vi "Drive Controller.vi"(8 "error in":errorcluster) -> ()   [LabVIEW 2019]
doc: "This VI executes continuously carrying out the current operation and responding to updates or new operation requests. It will often contain the timing or control code that is difficult to place directly in TeleOp. This VI generally opens all sensors and motors and isolates the rest of the robot code from knowing implementation details of how the operations are carried out."
uses:
  <vilib>/Rock Robotics/WPI/Framework/Completion Status.ctl
  Drive Setpoints.ctl
  Drive Operations.ctl
  <vilib>/Rock Robotics/WPI/ThirdParty/Phoenix-LabVIEW/Motor Controller/Controls/CTRE_Phoenix_MotorControl_ControlMode.ctl
  <vilib>/Rock Robotics/WPI/ThirdParty/Phoenix-LabVIEW/Motor Controller/Get/CTRE_Phoenix_MotorController_GetQuadratureData.vi
  <vilib>/Rock Robotics/WPI/SafetyOutput/WPI_SafetyOutputConfigMenu.ctl
  <vilib>/Rock Robotics/WPI/ThirdParty/Phoenix-LabVIEW/Motor Controller/Get/CTRE_Phoenix_MotorController_GetSelectedSensorData.vi
  <vilib>/Rock Robotics/WPI/RobotDrive/WPI_RobotDriveOpen2MotorWithExistingMotors.vi
panel:
  out "Analog Position 2":dbl
  out "Iterations":i32
  out "Analog Position":dbl
  in  "Interactive Values":T1
  in  "Buttons":cluster{"Execute Cmd":bool, "Abort Cmd":bool}
  out "Command Timing":cluster{"Start Time (ms)":u32, "Iterations":i32}
  out "Status":T3
  out "Current\nCmd":string
  # "Tip: The graph shows the motor setpoints. It may also be helpful to observe inputs and sensor values.\nYou may also want to display tuning or debugging controls."
  # "Interactive Command: You may fill in the settings for a command\nand schedule it with the Execute button. You can observe and abort\nany command while fine tuning the code for the controller."
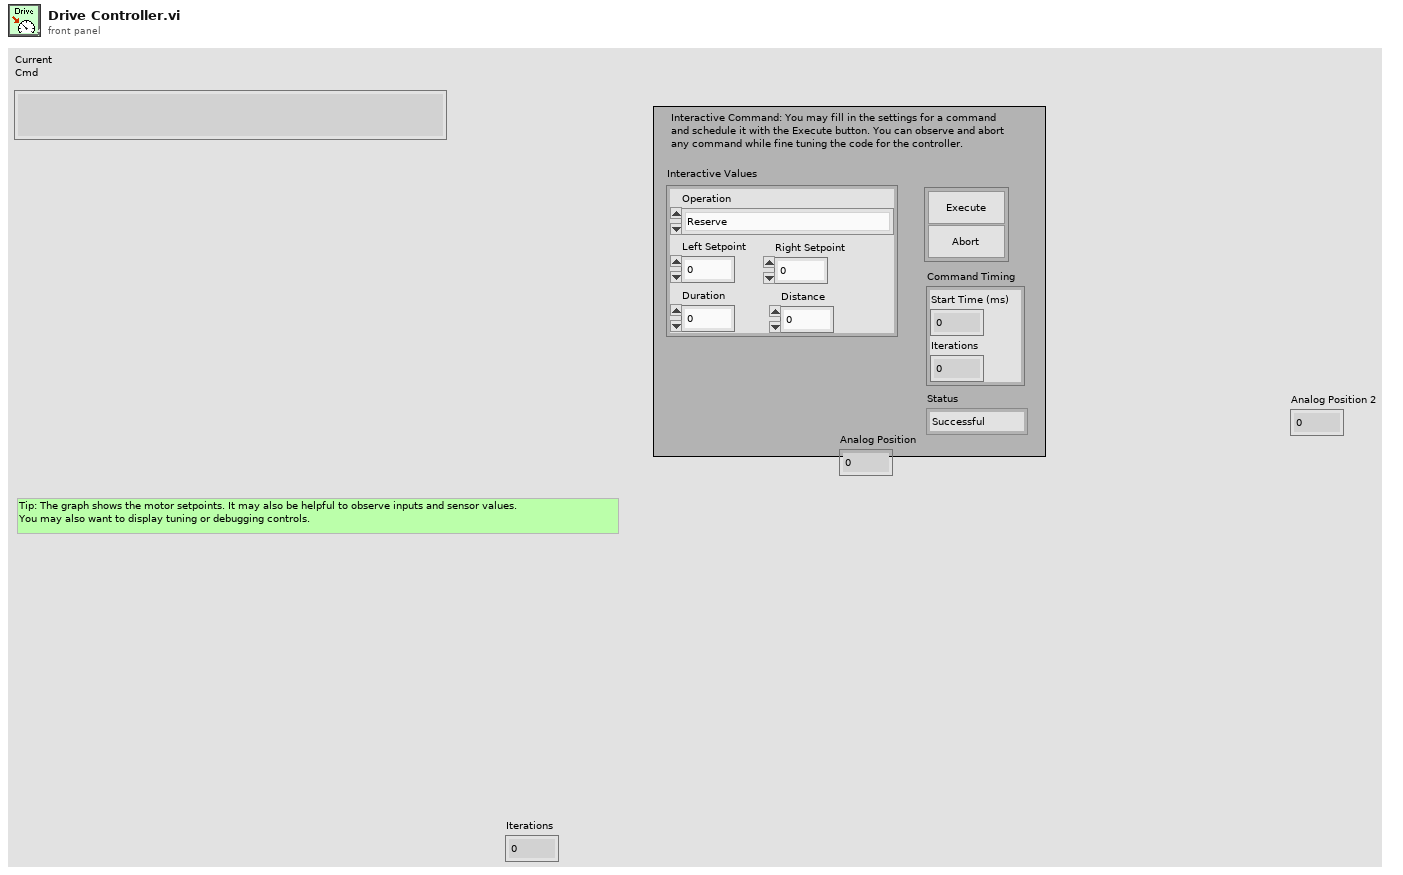
[diagram p1: front panel]
types:
  T1 = typedef "Drive Setpoints.ctl" = cluster{"Operation":T2, "Left Setpoint":dbl, "Right Setpoint":dbl, "Duration":dbl, "Distance":dbl}
  T2 = typedef "Drive Operations.ctl" = enum16{"Reserve", "Read Current", "Immediate", "Drive for Time", "Drive for Distance", "Turn angle"}
  T3 = typedef "Completion Status.ctl" = enum16{"Successful", "Aborted", "Incomplete"}
  T4 = typedef "WPI_SafetyOutputConfigMenu.ctl" = enum16{"Enable", "Disable"}
  T5 = typedef "WPI_MotorControlDeviceRef.ctl" = cluster{"DeviceStatus":errorcluster, "Type":T6, "PWM":cluster{"PWM Channel":T7, "DeadBand":T8}, "CAN":cluster{"Device Number":u8, "SetOutput VI Ref":variant, "GetOutput VI Ref":variant, "Enable VI Ref":variant, "Disable VI Ref":variant, "Data":variant}, "Invert":bool, "DIO PWM":cluster{"PWM \"Enable\" Channel":T7, "DIOChannel":T9, "PWM Rate":dbl}}
  T6 = typedef "WPI_MotorControlType.ctl" = enum16{"PWM", "CAN", "DIO PWM"}
  T7 = typedef "FPGA_DIOPWMChannel.ctl" = enum8{"PWM 0", "PWM 1", "PWM 2", "PWM 3", "PWM 4", "PWM 5", "PWM 6", "PWM 7", "PWM 8", "PWM 9", "PWM MXP 0", "PWM MXP 1", "PWM MXP 2", "PWM MXP 3", "PWM MXP 4", "PWM MXP 5", "PWM MXP 6", "PWM MXP 7", "PWM MXP 8", "PWM MXP 9", "Invalid"}
  T8 = typedef "WPI_PWMDeadband.ctl" = cluster{"Name":string, "maxPositivePwm":i32, "minPositivePwm":i32, "centerPwm":i32, "maxNegativePwm":i32, "minNegativePwm":i32, "angularRange":u16}
  T9 = typedef "FPGA_DIOChannel.ctl" = enum8{"DIO 0", "DIO 1", "DIO 2", "DIO 3", "DIO 4", "DIO 5", "DIO 6", "DIO 7", "DIO 8", "DIO 9", "DIO MXP 0", "DIO MXP 1", "DIO MXP 2", "DIO MXP 3", "DIO MXP 4", "DIO MXP 5", "DIO MXP 6", "DIO MXP 7", "DIO MXP 8", "DIO MXP 9", "DIO MXP 10", "DIO MXP 11", "DIO MXP 12", "DIO MXP 13", "DIO MXP 14", "DIO MXP 15", "SPI Port CS1", "SPI Port CS2", "SPI Port CS3", "SPI Port MISO", "SPI Port MOSI", "Invalid"}
  T10 = typedef "WPI_RobotDriveDevRef.ctl" = cluster{"DevStatus":errorcluster, "Motors[]":T5[], "Square Inputs":bool, "Max Output":dbl}
  T11 = enum16{"FollowerType_PercentOutput", "FollowerType_AuxOutput1"}
  T12 = typedef "Command Status Info.ctl" = cluster{"Name":string, "Status":T3, "notifier out":T13}
  T13 = typedef "Completion Notifier.ctl" = refnum<notifier>
  T14 = cluster{"SubSystem Data":T1, cluster{"Start Time (ms)":u32, "Iterations":i32}, cluster{"Command Info":T12, "Description":string, "Default Command":T1, "queue out":refnum<queue>, "Subsystem Name":string}}
  T15 = typedef "CTRE_Phoenix_MotorControl_ControlMode.ctl" = u16
  T16 = cluster{"SubSystem Data":T1, cluster{"Start Time (ms)":u32, "Iterations":i32}, "Default Command Arguments":cluster{"Command Info":T12, "Description":string, "Default Command":T1, "queue out":refnum<queue>, "Subsystem Name":string}}
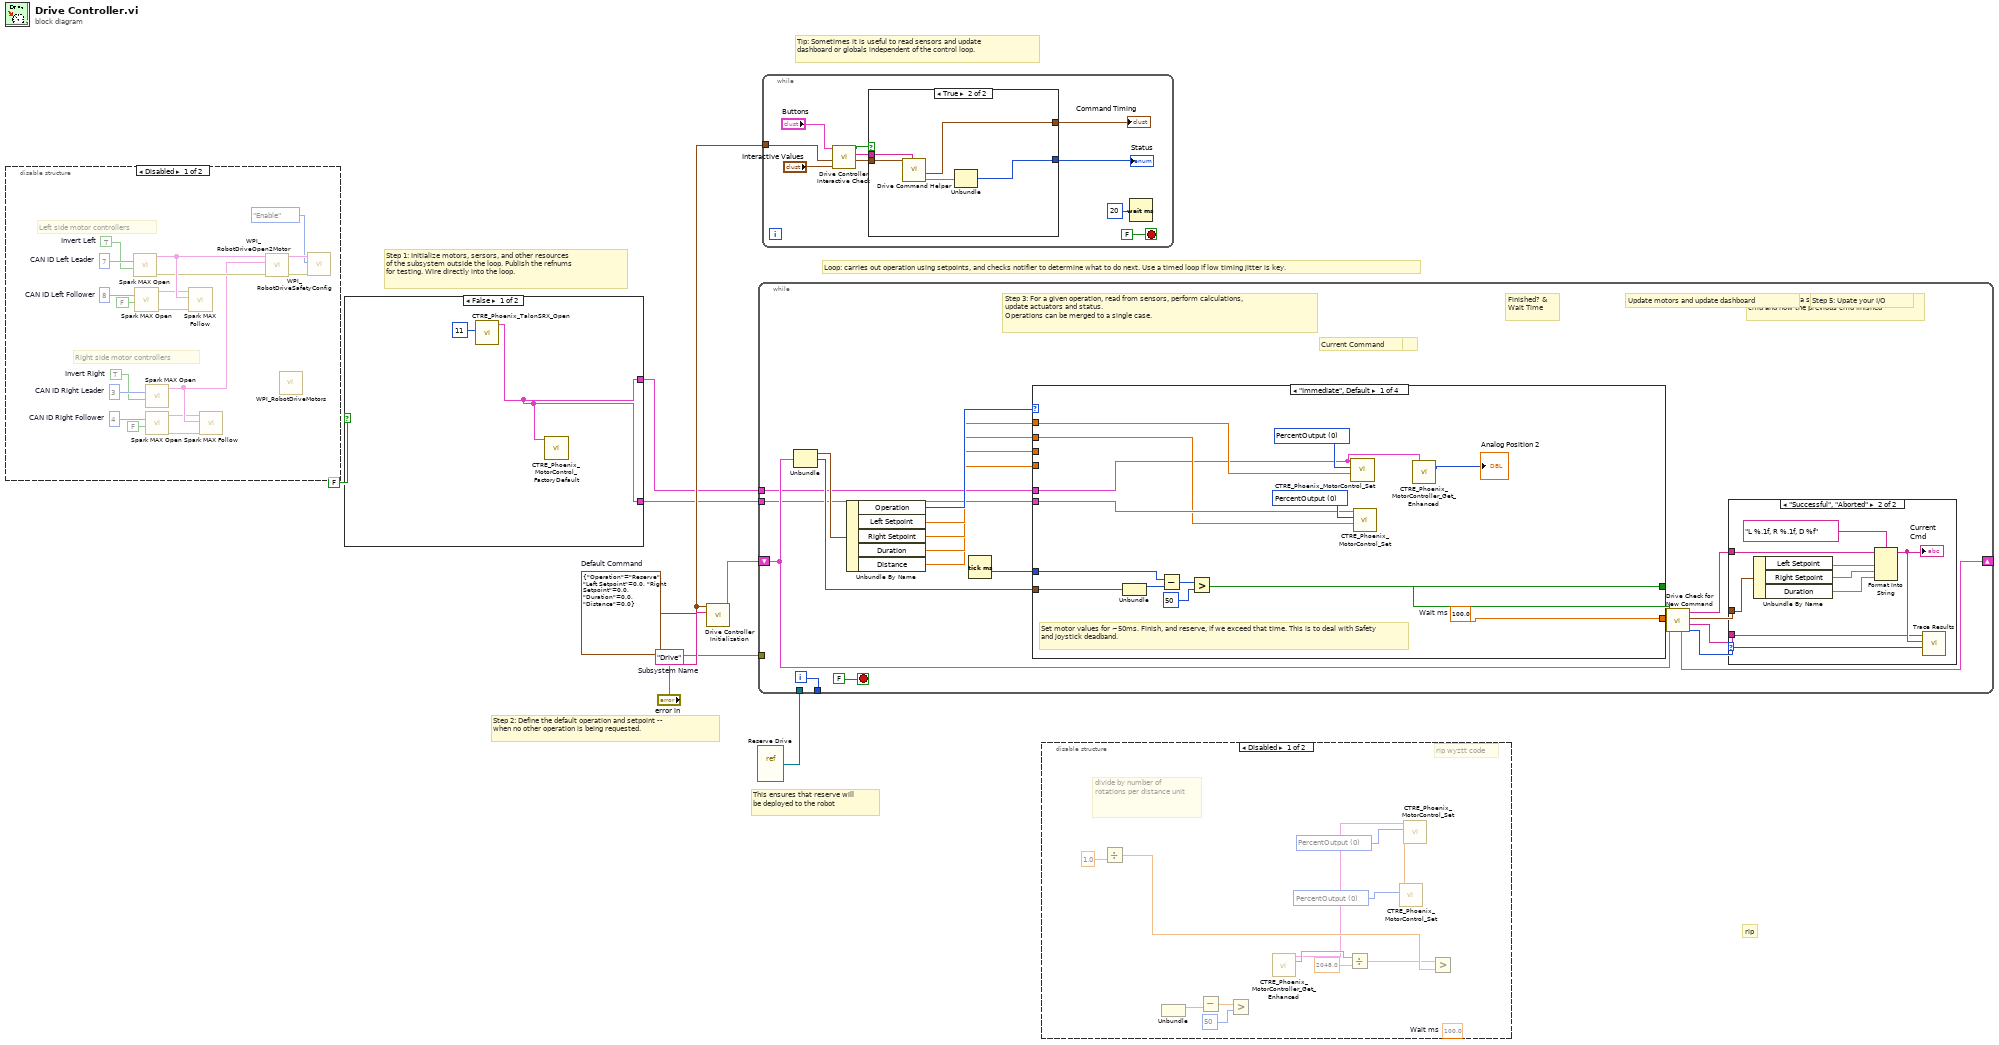
[diagram p0: block diagram]
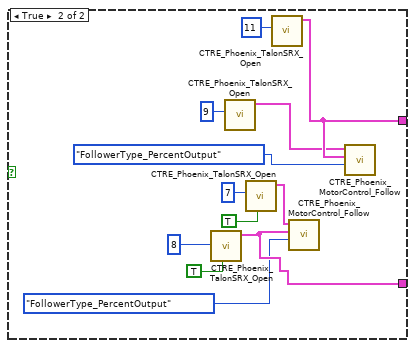
[diagram p2: hidden frame]
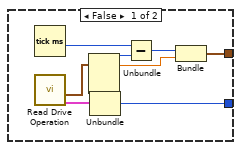
[diagram p5: hidden frame]
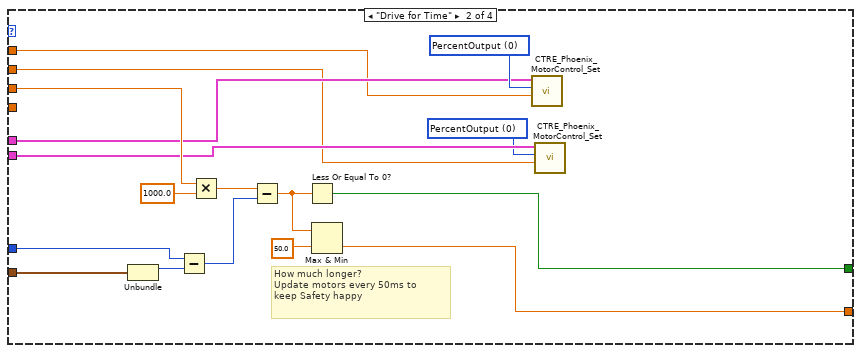
[diagram p7: hidden frame]
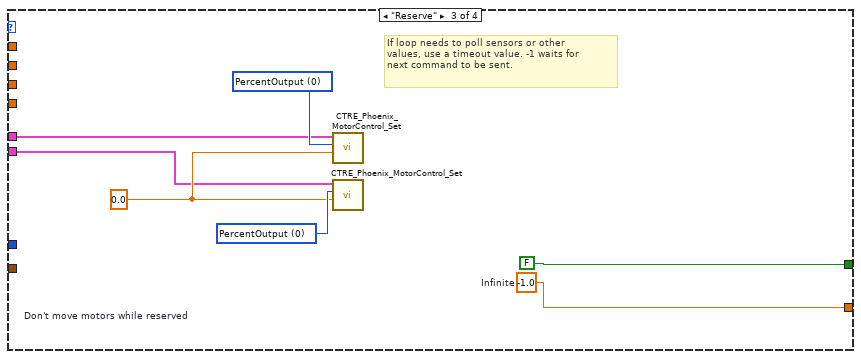
[diagram p8: hidden frame]
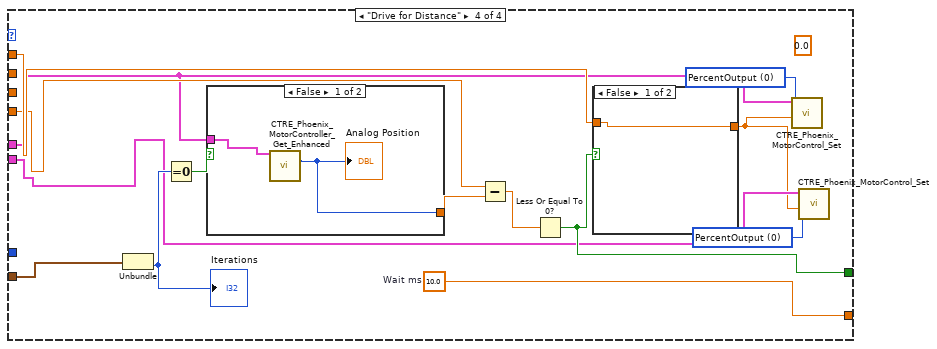
[diagram p9: hidden frame]
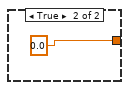
[diagram p10: hidden frame]
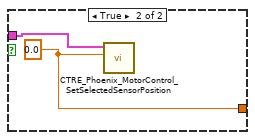
[diagram p11: hidden frame]
diagram:
  w4 = T1 {"Operation"=enum."Reserve", "Left Setpoint"=0.0, "Right Setpoint"=0.0, "Duration"=0.0, "Distance"=0.0}  # Default Command
  w8 = "Drive"  # Subsystem Name
  # "rip"
  # "This ensures that reserve will\nbe deployed to the robot"
  # "Tip: Sometimes it is useful to read sensors and update\ndashboard or globals independent of the control loop."
  # "Step 2: Define the default operation and setpoint --\nwhen no other operation is being requested."
  # "Step 1: Initialize motors, sersors, and other resources\nof the subsystem outside the loop. Publish the refnums\nfor testing. Wire directly into the loop."
  # "Loop: carries out operation using setpoints, and checks notifier to determine what to do next. Use a timed loop if low timing jitter is key."
  n1 = disable-structure shown="Disabled" {
    frame Disabled {
      w15 = TRUE  # Invert Left
      w14 = TRUE  # Invert Right
      w20 = u8 3  # CAN ID Right Leader
      w19 = u8 4  # CAN ID Right Follower
      w26 = u8 7  # CAN ID Left Leader
      w27 = u8 8  # CAN ID Left Follower
      # "Right side motor controllers"
      # "Left side motor controllers"
      n2 = call <vilib>:"Spark MAX Open.vi"("Invert"=w15, "Device Number"=w26) -> ("error out"=w24:errorcluster, "MotorControlDeviceRef"=w25:T5)  [unwired: 8 in]
      n3 = call <vilib>:"Spark MAX Open.vi"("Invert"=FALSE, "Device Number"=w27) -> ("error out"=w22:errorcluster, "MotorControlDeviceRef"=w23:T5)  [unwired: 8 in]
      n4 = call <vilib>:"Spark MAX Open.vi"("Invert"=w14, "Device Number"=w20) -> ("MotorControlDeviceRef"=w11:T5)  [unwired: 8 in, 1 out]
      n5 = call <vilib>:"Spark MAX Open.vi"("Invert"=FALSE, "Device Number"=w19) -> ("error out"=w21:errorcluster, "MotorControlDeviceRef"=w9:T5)  [unwired: 8 in]
      n6 = call <vilib>:"Spark MAX Follow.vi"("error in (no error)"=w22, "Master Controller"=w25, "MotorControlDeviceRef"=w23) -> ()  [unwired: 7 in, 2 out]
      n7 = call <vilib>:"Spark MAX Follow.vi"("error in (no error)"=w21, "Master Controller"=w11, "MotorControlDeviceRef"=w9) -> ()  [unwired: 7 in, 2 out]
      n8 = call-poly <vilib>:"WPI_RobotDriveOpen2Motor.vi"("error in (no error)"=w24, "Right Motor Dev Ref"=w11, "Left Motor Dev Ref"=w25) -> ("error out"=w17:errorcluster, "RobotDriveDevRef"=w18:T10)  [unwired: 7 in]
      n9 = call <vilib>:"WPI_RobotDriveMotors.vi"() -> ()  [unwired: 4 in, 8 out]
      n10 = call <vilib>:"WPI_RobotDriveSafetyConfig.vi"("error in (no error)"=w17, "mode"=WPI_SafetyOutputConfigMenu."Enable", "RobotDriveDevRef"=w18) -> ("RobotDriveDevRef"=w10:T10)  [unwired: 7 in, 1 out]
    }
    frame Enabled {
    }
  }
  n11 = case shown="False" FALSE {
    tunnel: [w28 w40] -> w3
    tunnel: [w28 w37] -> w2
    frame False {
      n12 = call <vilib>:"CTRE_Phoenix_TalonSRX_Open.vi"("Device Number"=u8 11) -> ("CAN Talon SRX Ref"=w28:T5)  [unwired: 9 in, 1 out]
      n13 = call <vilib>:"CTRE_Phoenix_MotorControl_FactoryDefault.vi"("PhoenixMotorControlDevRef"=w28) -> ()  [unwired: 9 in, 2 out]
    }
    frame True {
      n14 = call <vilib>:"CTRE_Phoenix_TalonSRX_Open.vi"("Invert"=TRUE, "Device Number"=u8 8) -> ("CAN Talon SRX Ref"=w37:T5)  [unwired: 8 in, 1 out]
      n15 = call <vilib>:"CTRE_Phoenix_TalonSRX_Open.vi"("Device Number"=u8 9) -> ("CAN Talon SRX Ref"=w39:T5)  [unwired: 9 in, 1 out]
      n16 = call <vilib>:"CTRE_Phoenix_TalonSRX_Open.vi"("Invert"=TRUE, "Device Number"=u8 7) -> ("CAN Talon SRX Ref"=w38:T5)  [unwired: 8 in, 1 out]
      n17 = call <vilib>:"CTRE_Phoenix_TalonSRX_Open.vi"("Device Number"=u8 11) -> ("CAN Talon SRX Ref"=w40:T5)  [unwired: 9 in, 1 out]
      n18 = call <vilib>:"CTRE_Phoenix_MotorControl_Follow.vi"("FollowerType"=T11."FollowerType_PercentOutput", "Master Controller to Follow"=w37, "PhoenixMotorControlDevRef"=w38) -> ()  [unwired: 7 in, 2 out]
      n19 = call <vilib>:"CTRE_Phoenix_MotorControl_Follow.vi"("FollowerType"=T11."FollowerType_PercentOutput", "Master Controller to Follow"=w40, "PhoenixMotorControlDevRef"=w39) -> ()  [unwired: 7 in, 2 out]
    }
  }
  n20 = call "Drive Controller Initialization.vi"("Subsystem Name"=w8, "Default Command"=w4) -> ("Current Command"=w6:T14)  [unwired: 9 in]
  n21 = vi-ref "Reserve Drive.vi"() -> (w5:refnum<vi>)
  n22 = while {
    shift-right: [w52] -> _
    shift-left: w6 -> [w45]
    tunnel: [w60] -> _
    tunnel: "error in" -> [_]
    tunnel: w5 -> [_]
    tunnel: w2 -> [w43]
    tunnel: w3 -> [w42]
    i -> [w60]
    stop <- FALSE stop-if-true
    # "Step 5: Upate your I/O"
    # "Step 4: Format a string to describe this\ncmd and how the previous cmd finished"
    # "Current Command"
    # "Update motors and update dashboard"
    # "Access Cmd setpoints"
    # "Finished? &\nWait Time"
    # "Step 3: For a given operation, read from sensors, perform calculations,\nupdate actuators and status.\nOperations can be merged to a single case."
    n23 = Unbundle(w45) -> ("SubSystem Data"=w59:T1, w46:cluster{"Start Time (ms)":u32, "Iterations":i32})  [unwired: 1 out]
    n24 = Unbundle By Name(w59) -> ("Operation"=w58:T2, "Left Setpoint"=w57:dbl, "Right Setpoint"=w56:dbl, "Duration"=w55:dbl, "Distance"=w44:dbl)
    n25 = Tick Count (ms)() -> (millisecond timer value=w54:u32)
    n26 = case shown="\"Immediate\", Default" w58 {
      tunnel: [w84 w91 w108 w115] -> w51
      tunnel: [w79 w96 FALSE ("ignore previous (F)") w114] -> w50
      tunnel: w46 -> [w78 w98 _ w116]
      tunnel: w57 -> [w74 w87 _ w118]
      tunnel: w56 -> [w73 w86 _ _]
      tunnel: w55 -> [_ w95 _ _]
      tunnel: w54 -> [w80 w94 _ _]
      tunnel: w44 -> [_ _ _ w117]
      tunnel: w43 -> [w75 w88 w102 w113]
      tunnel: w42 -> [w72 w89 w103 w109]
      frame "Immediate", Default {
        w76 = T15 0 items=["PercentOutput"=0, "Position"=1, "Velocity"=2, "Current"=3, "Follower"=5, "MotionProfile"=6, "MotionMagic"=7, "MotionProfileArc"=10, "Disabled"=15] ("Control Mode")
        w77 = T15 0 items=["PercentOutput"=0, "Position"=1, "Velocity"=2, "Current"=3, "Follower"=5, "MotionProfile"=6, "MotionMagic"=7, "MotionProfileArc"=10, "Disabled"=15] ("Control Mode")
        w84 = 100.0  # Wait ms
        # "Set motor values for ~50ms. Finish, and reserve, if we exceed that time. This is to deal with Safety and joystick deadband."
        n27 = Unbundle(w78) -> ("Start Time (ms)"=w81:u32)  [unwired: 1 out]
        n28 = Subtract(x=w80, y=w81) -> (x-y=w82:u32)
        n29 = Greater?(x=w82, y=u8 50 ("Left Motor")) -> (0:w79:bool)
        n30 = call <vilib>:"CTRE_Phoenix_MotorControl_Set.vi"("Output"=w74, "Control Mode"=w77, "PhoenixMotorControlDevRef"=w72) -> ()  [unwired: 7 in, 2 out]
        n31 = call <vilib>:"CTRE_Phoenix_MotorControl_Set.vi"("Output"=w73, "Control Mode"=w76, "PhoenixMotorControlDevRef"=w75) -> ()  [unwired: 7 in, 2 out]
        n32 = call-poly <vilib>:"CTRE_Phoenix_MotorController_Get_Enhanced.vi"("PhoenixMotorControlDevRef"=w72) -> ("Quadrature Position"=→"Analog Position 2":i32)  [unwired: 11 in, 3 out]
      }
      frame "Drive for Time" {
        w85 = T15 0 items=["PercentOutput"=0, "Position"=1, "Velocity"=2, "Current"=3, "Follower"=5, "MotionProfile"=6, "MotionMagic"=7, "MotionProfileArc"=10, "Disabled"=15] ("Control Mode")
        w90 = T15 0 items=["PercentOutput"=0, "Position"=1, "Velocity"=2, "Current"=3, "Follower"=5, "MotionProfile"=6, "MotionMagic"=7, "MotionProfileArc"=10, "Disabled"=15] ("Control Mode")
        # "How much longer?\nUpdate motors every 50ms to\nkeep Safety happy"
        n33 = Unbundle(w98) -> ("Start Time (ms)"=w97:u32)  [unwired: 1 out]
        n34 = Subtract(x=w94, y=w97) -> (x-y=w101:u32)
        n35 = Multiply(x=w95, y=1000.0) -> (x*y=w100:dbl)
        n36 = Subtract(x=w100, y=w101) -> (x-y=w93:dbl)
        n37 = Less Or Equal To 0?(x=w93) -> (x <= 0?=w96:bool)
        n38 = Max & Min(x=w93, y=50.0) -> (min(x,y)=w91:dbl)  [unwired: 1 out]
        n39 = call <vilib>:"CTRE_Phoenix_MotorControl_Set.vi"("Output"=w87, "Control Mode"=w90, "PhoenixMotorControlDevRef"=w89) -> ()  [unwired: 7 in, 2 out]
        n40 = call <vilib>:"CTRE_Phoenix_MotorControl_Set.vi"("Output"=w86, "Control Mode"=w85, "PhoenixMotorControlDevRef"=w88) -> ()  [unwired: 7 in, 2 out]
      }
      frame "Reserve" {
        w105 = T15 0 items=["PercentOutput"=0, "Position"=1, "Velocity"=2, "Current"=3, "Follower"=5, "MotionProfile"=6, "MotionMagic"=7, "MotionProfileArc"=10, "Disabled"=15] ("Control Mode")
        w106 = T15 0 items=["PercentOutput"=0, "Position"=1, "Velocity"=2, "Current"=3, "Follower"=5, "MotionProfile"=6, "MotionMagic"=7, "MotionProfileArc"=10, "Disabled"=15] ("Control Mode")
        w104 = 0.0  # Don't move motors while reserved
        w108 = -1.0  # Infinite
        # "If loop needs to poll sensors or other\nvalues, use a timeout value. -1 waits for\nnext command to be sent."
        n41 = call <vilib>:"CTRE_Phoenix_MotorControl_Set.vi"("Output"=w104, "Control Mode"=w106, "PhoenixMotorControlDevRef"=w103) -> ()  [unwired: 7 in, 2 out]
        n42 = call <vilib>:"CTRE_Phoenix_MotorControl_Set.vi"("Output"=w104, "Control Mode"=w105, "PhoenixMotorControlDevRef"=w102) -> ()  [unwired: 7 in, 2 out]
      }
      frame "Drive for Distance" {
        w110 = T15 0 items=["PercentOutput"=0, "Position"=1, "Velocity"=2, "Current"=3, "Follower"=5, "MotionProfile"=6, "MotionMagic"=7, "MotionProfileArc"=10, "Disabled"=15] ("Control Mode")
        w111 = T15 0 items=["PercentOutput"=0, "Position"=1, "Velocity"=2, "Current"=3, "Follower"=5, "MotionProfile"=6, "MotionMagic"=7, "MotionProfileArc"=10, "Disabled"=15] ("Control Mode")
        (unwired) 0.0 ("f")
        w115 = 10.0  # Wait ms
        n43 = Unbundle(w116) -> ("Iterations"=w122:i32)  [unwired: 1 out]
        "Iterations" <- w122
        n44 = Equal To 0?(x=w122) -> (x = 0?=w121:bool)
        n45 = case shown="False" w121 {
          tunnel: w109 -> [w126 w128]
          tunnel: [w125 w127] -> w120
          frame False {
            n46 = call-poly <vilib>:"CTRE_Phoenix_MotorController_Get_Enhanced.vi"("PhoenixMotorControlDevRef"=w126) -> ("Quadrature Position"=w125:i32)  [unwired: 11 in, 3 out]
            "Analog Position" <- w125
          }
          frame True {
            w127 = 0.0 ("Position")
            n47 = call <vilib>:"CTRE_Phoenix_MotorControl_SetSelectedSensorPosition.vi"("New Sensor Position"=w127, "PhoenixMotorControlDevRef"=w128) -> ()  [unwired: 8 in, 2 out]
          }
        }
        n48 = Subtract(x=w117, y=w120) -> (x-y=w119:dbl)
        n49 = Less Or Equal To 0?(x=w119) -> (x <= 0?=w114:bool)
        n50 = case shown="False" w114 {
          tunnel: [w123 0.0 ("Setpoint")] -> w112
          tunnel: w118 -> [w123 _]
          frame False {
          }
          frame True {
          }
        }
        n51 = call <vilib>:"CTRE_Phoenix_MotorControl_Set.vi"("Output"=w112, "Control Mode"=w111, "PhoenixMotorControlDevRef"=w109) -> ()  [unwired: 7 in, 2 out]
        n52 = call <vilib>:"CTRE_Phoenix_MotorControl_Set.vi"("Output"=w112, "Control Mode"=w110, "PhoenixMotorControlDevRef"=w113) -> ()  [unwired: 7 in, 2 out]
      }
    }
    n53 = call "Drive Check for New Command.vi"("input cluster"=w45, "Wait time (ms)"=w51, "Finished?"=w50) -> ("Completion"=w53:T3, "Subsystem Name"=w47:string, "Current Command"=w48:T1, "Initial Trace String"=w49:string, "Next Command"=w52:T16)  [unwired: 4 in]
    n54 = case shown="\"Successful\", \"Aborted\"" w53 {
      selector: w53 -> [_ w70]
      tunnel: w49 -> [_ w65]
      tunnel: w48 -> [_ w66]
      tunnel: w47 -> [_ w62]
      frame "Incomplete", Default {
        # "Continuing current command"
      }
      frame "Successful", "Aborted" {
        # "Report and setup for next command"
        n55 = Unbundle By Name(w66) -> ("Left Setpoint"=w68:dbl, "Right Setpoint"=w69:dbl, "Duration"=w63:dbl)
        n56 = Format Into String(format string="L %.1f, R %.1f, D %f", initial string=w65, w68, w69, w63) -> (resulting string=w64:string)  [unwired: 1 in, 1 out]
        "Current\nCmd" <- w64
        n57 = call <vilib>:"Trace Results.vi"("Status of previous command"=w70, "Description"=w64, "Subsystem"=w62) -> ()  [unwired: 9 in]
      }
    }
  }
  n58 = while {
    tunnel: w4 -> [w130]
    stop <- FALSE stop-if-true
    n59 = call "Drive Controller Interactive Check.vi"("Interactive Command In"="Interactive Values", "Default Command"=w130, "Buttons"="Buttons") -> ("Interactive Command Out"=w132:T1, "Trace String"=w133:string, "Schedule"=w134:bool)  [unwired: 6 in]
    n60 = case shown="True" w134 {
      tunnel: [w143 w151] -> w135
      tunnel: [w142 w147] -> w136
      tunnel: w133 -> [_ w149]
      tunnel: w132 -> [_ w148]
      frame False {
        n61 = Tick Count (ms)() -> (millisecond timer value=w146:u32)
        n62 = call "Read Drive Operation.vi"() -> ("Command Info"=w140:T12, "SubSystem Data"=w139:T1)  [unwired: 9 in, 1 out]
        n63 = Unbundle(w139) -> ("Operation"=w144:T2, "Left Setpoint"=w141:dbl)  [unwired: 3 out]
        n64 = Unbundle(w140) -> ("Status"=w143:T3)  [unwired: 2 out]
        n65 = Subtract(x=w146, y=w144) -> (x-y=w145:u32)
        n66 = Bundle(w145, "Left Setpoint"=w141) -> (w142:cluster{u32, "Left Setpoint":dbl})  [unwired: 1 in]
      }
      frame True {
        n67 = call "Drive Command Helper.vi"("Description"=w149, "SubSystem Data"=w148) -> ("Command Info Out"=w150:T12, "Command Timing"=w147:cluster{"Start Time (ms)":u32, "Iterations":i32})  [unwired: 7 in, 1 out]
        n68 = Unbundle(w150) -> ("Status"=w151:T3)  [unwired: 2 out]
      }
    }
    "Status" <- w135
    "Command Timing" <- w136
    n69 = Wait (ms)(milliseconds to wait=u32 20) -> ()  [unwired: 1 out]
  }
  n70 = disable-structure shown="Disabled" {
    frame Disabled {
      w156 = T15 0 items=["PercentOutput"=0, "Position"=1, "Velocity"=2, "Current"=3, "Follower"=5, "MotionProfile"=6, "MotionMagic"=7, "MotionProfileArc"=10, "Disabled"=15] ("Control Mode")
      w159 = T15 0 items=["PercentOutput"=0, "Position"=1, "Velocity"=2, "Current"=3, "Follower"=5, "MotionProfile"=6, "MotionMagic"=7, "MotionProfileArc"=10, "Disabled"=15] ("Control Mode")
      w164 = 100.0  # Wait ms
      # "rip wyztt code"
      # "divide by number of rotations per distance unit"
      n71 = Divide(y=1.0) -> (x/y=w168:dbl)  [unwired: 1 in]
      n72 = Unbundle() -> (w163:cluster{"Start Time (ms)":u32, "Iterations":i32}, "Start Time (ms)"=w162)  [unwired: 1 out]
      n73 = Subtract(y=w162) -> (x=w161:dbl, x-y=w165:dbl)
      n74 = Greater?(x=w165, y=u8 50 ("Left Motor")) -> ()  [unwired: 1 out]
      n75 = call <vilib>:"CTRE_Phoenix_MotorControl_Set.vi"("Control Mode"=w156) -> ("Output"=w160:dbl, "PhoenixMotorControlDevRef"=w153:T5)  [unwired: 7 in, 2 out]
      n76 = call-poly <vilib>:"CTRE_Phoenix_MotorController_Get_Enhanced.vi"("PhoenixMotorControlDevRef"=w153) -> ("Position (Raw Sensor Units)"=w155:i32)  [unwired: 11 in, 3 out]
      n77 = Divide(x=w155, y=2048.0) -> (x/y=w158:dbl)
      n78 = call <vilib>:"CTRE_Phoenix_MotorControl_Set.vi"("Output"=w160, "Control Mode"=w159) -> ("PhoenixMotorControlDevRef"=w152:T5)  [unwired: 7 in, 2 out]
      n79 = Greater?(x=w158, y=w168) -> (0:w154:bool)
    }
    frame Enabled {
    }
  }
